vi "Configure Device.vi"(8 "error in":errorcluster, 11 "Alicat Device In":refnum<class "Alicat Device.lvclass">) -> (0 "error out":errorcluster, 3 "Alicat Device Out":refnum<class "Alicat Device.lvclass">, 4 "SP":dbl, 5 "Settable?":bool)   [LabVIEW 2014, in "Alicat Lib.lvlib" / "Alicat Device.lvclass"]
doc: "Configure the serial port for communication with the Alicat devices. We will create new Alicat objects based upon an input array of addresses. If an address is no good, then we will delete the session reference and move onto the next address. We determine if the session is good by sending a request for data to the device until the device \"wakes up\" and responds properly. If the device does not repsond properly, then set the boolean property <b>Active</b> to alert potential callers that this instantiation is non-communicative.\n\nAlthough the caller can configure the port with the desired serial and message settings, the default settings should be sufficient for most applications."
uses:
  Alicat Device.lvclass
  reusable/Session APIs/Serial/Serial Session.lvclass
  Data/Alicat Data.lvclass
  Configurable Device/Configurable Device.lvclass/Configurable Device.ctl
  reusable/Data/Data.lvclass/Data.ctl
  Data/Alicat Data.lvclass/Alicat Data.ctl
  Alicat Device.lvclass/Alicat Device.ctl
  reusable/Session APIs/File Access/Config Data/Config Data.lvclass/Config Data.ctl
  Configurable Device/Accessors/Write label.vi
  Accessors/Read Session Handle.vi
  Configurable Device/Read controller_.vi
  Accessors/Write Session Handle.vi
  Configurable Device/Accessors/Write type.vi
  reusable/Data/Write Data ID.vi
  Data/Accessors/Write ID.vi
  Configurable Device/Read Handle.vi
  Configurable Device/Read Log Session.vi
  <vilib>/Utility/config.llb/Read Key (String).vi
  <vilib>/Utility/config.llb/Read Key (Double).vi
  Configurable Device/Configurable Device.lvclass
  reusable/Session APIs/File Access/Config Data/Config Data.lvclass
  <userlib>/_Session Fwk/Session - Root.lvclass
  <vilib>/ErrorRing/Error Ring.xnode
  <vilib>/Utility/config.llb/NI_LVConfig.lvlib
  reusable/Session APIs/Session Log/System Log.lvclass
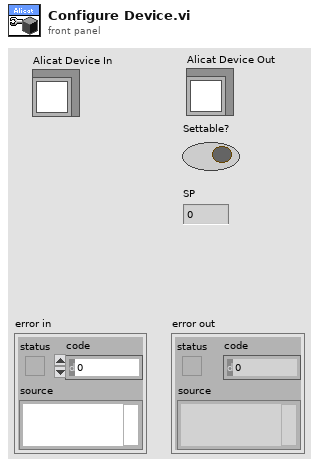
[diagram p1: front panel]
types:
  T1 = typedef "Serial Session.lvclass/Session Handle.ctl" = refnum<data-value>
  T2 = typedef "Config Data.lvclass/Config Session.ctl" = refnum<data-value>
  T3 = typedef "Session - Root.lvclass/Session Handle.ctl" = refnum<data-value>
  T4 = typedef "NI_LVConfig.lvlib/Config Data RefNum.ctl" = refnum<k1>
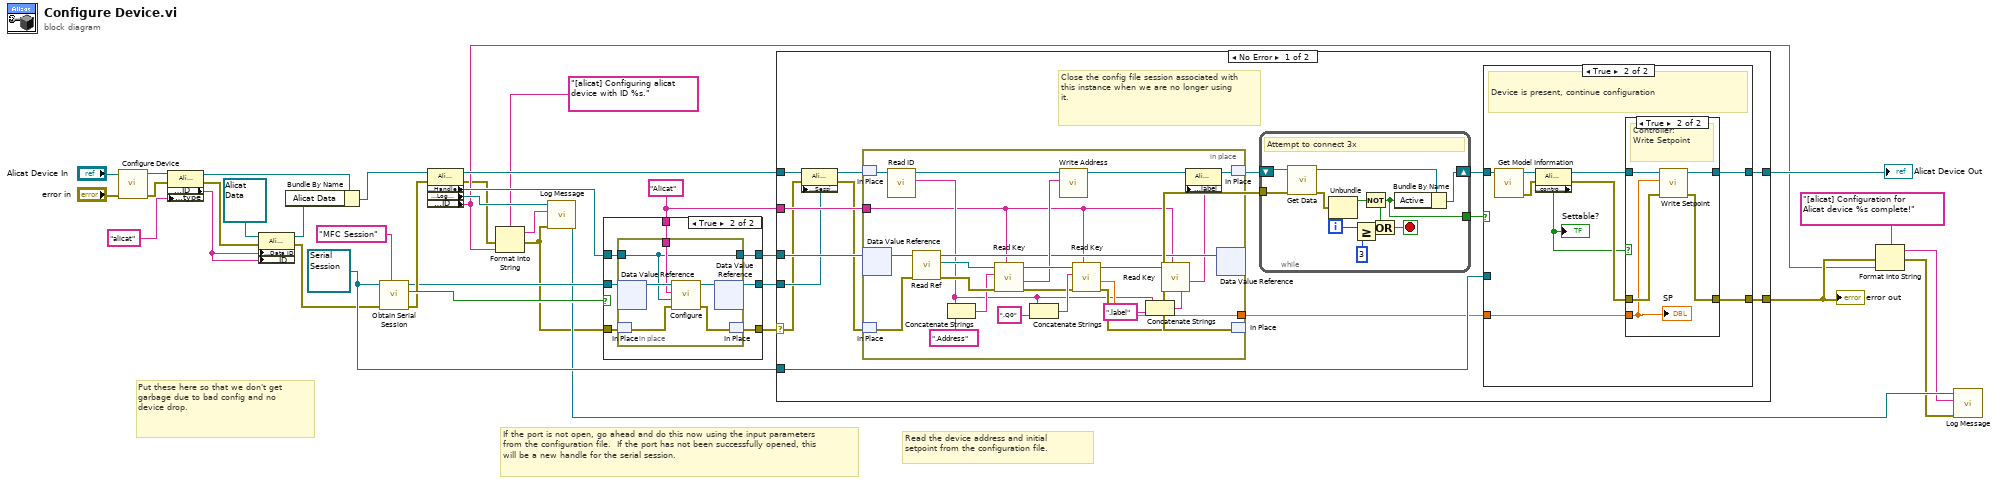
[diagram p0: block diagram]
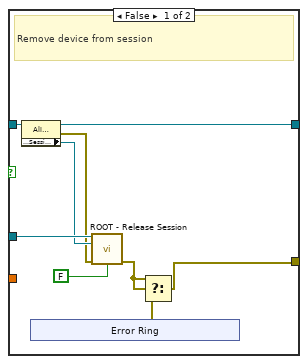
[diagram p2: hidden frame]
diagram:
  w28 = refnum<class "Serial Session.lvclass"> refnum ("Serial Session in")
  w30 = "Alicat" ("section")
  # "Put these here so that we don't get garbage due to bad config and no device drop."
  # "If the port is not open, go ahead and do this now using the input parameters from the configuration file.  If the port has not been successfully opened, this will be a new handle for the serial session."
  # "Read the device address and initial setpoint from the configuration file."
  n1 = call-parent "Configure Device.vi"("error in"="error in", "Device in"="Alicat Device In") -> ("error out"=w2:errorcluster, "Device out"=w3:refnum<class "Alicat Device.lvclass">)  [unwired: 6 in, 2 out]
  n2 = property class="Alicat Device"(reference=w3, error in=w2, "Accessors:type"="alicat" ("type")) -> (reference out=w12:refnum<class "Alicat Device.lvclass">, error out=w9:errorcluster, "Accessors:ID"=w13:string)
  n3 = property class="Alicat Data"(reference=refnum<class "Alicat Data.lvclass"> refnum ("Alicat Lib.lvlib:Alicat Data"), error in=w9, "Accessors:Data ID"=w13, "Accessors:ID"=w13) -> (reference out=w10:refnum<class "Alicat Data.lvclass">, error out=w8:errorcluster)
  n4 = Bundle By Name(cluster=w12, "Alicat Data"=w10) -> (w11:refnum<class "Alicat Device.lvclass">)
  n5 = call "Obtain Serial Session.vi"("Session Name ()"="MFC Session", "error in"=w8, "Serial Session in"=w28) -> ("error out"=w32:errorcluster, "created new?"=w35:bool, "hSerial"=w29:T1)  [unwired: 6 in]
  n6 = property class="Alicat Device"(reference=w11, error in=w32) -> (reference out=w27:refnum<class "Alicat Device.lvclass">, error out=w7:errorcluster, "Accessors:Handle"=w33:T2, "Accessors:Log Session"=w23:T3, "Accessors:ID"=w15:string)
  n7 = Format Into String(format string="[alicat] Configuring alicat device with ID %s.", error in=w7, w15) -> (resulting string=w21:string, error out=w6:errorcluster)  [unwired: 1 in]
  n8 = call "Log Message.vi"("error in"=w6, "MSG In"=w21, "session in"=w23) -> ("session out"=w20:T3)  [unwired: 7 in, 1 out]
  n9 = case shown="True" w35 {
    tunnel: w29 -> [w38 w45]
    tunnel: w6 -> [w37 w41]
    tunnel: [w38 w44] -> w26
    tunnel: [w37 w43] -> w25
    tunnel: w33 -> [w36 w42]
    tunnel: [w36 w40] -> w31
    tunnel: w30 -> [_ w39]
    frame False {
    }
    frame True {
      n10 = in-place {
        in-place-border: w42 -> [w46]
        in-place-border: w39 -> [w47]
        in-place-border: [w46] -> w40
        n11 = in-place-dvr #1(w45) -> (w51:refnum<class "Serial Session.lvclass">)  [unwired: 1 out]
        n12 = in-place-match #2(w41) -> (w50:errorcluster)
        n13 = call "Configure.vi"("error in"=w50, "Config Handle"=w46, "section"=w47, "Serial Session in"=w51) -> ("error out"=w49:errorcluster, "Serial Session out"=w48:refnum<class "Serial Session.lvclass">)  [unwired: 6 in]
        n14 = in-place-dvr #1(w48) -> (w44:T1)  [unwired: 1 out]
        n15 = in-place-match #2(w49) -> (w43:errorcluster)
      }
    }
  }
  n16 = case shown="No Error" w25 {
    selector: w25 -> [w54 w128]
    tunnel: w31 -> [w66 _]
    tunnel: w30 -> [w65 _]
    tunnel: w28 -> [w64 _]
    tunnel: [w62 w128] -> w16
    tunnel: [w59 w129] -> w24
    tunnel: w27 -> [w58 w129]
    tunnel: w26 -> [w56 _]
    frame No Error {
      # "Close the config file session associated with this instance when we are no longer using it."
      n17 = property class="Alicat Device"(reference=w58, error in=w54, "Accessors:Session Handle"=w56) -> (reference out=w57:refnum<class "Alicat Device.lvclass">, error out=w55:errorcluster)
      n18 = in-place {
        in-place-border: w65 -> [w104]
        in-place-border: [w116] -> w60
        n19 = in-place-match #3(w57) -> (w114:refnum<class "Alicat Device.lvclass">)
        n20 = in-place-dvr #4(w66) -> (w127:refnum<class "Config Data.lvclass">)  [unwired: 1 out]
        n21 = in-place-match #5(w55) -> (w126:errorcluster)
        n22 = call "Read ID.vi"("Configurable Device in"=w114) -> ("ID"=w107:string, "Configurable Device out"=w113:refnum<class "Alicat Device.lvclass">)  [unwired: 8 in, 1 out]
        n23 = call "Read Ref.vi"("error in"=w126, "Config Data in"=w127) -> ("error out"=w124:errorcluster, "config data"=w125:T4, "Config Data out"=w115:refnum<class "Config Data.lvclass">)  [unwired: 7 in]
        n24 = Concatenate Strings(w107, ".Address" ("string")) -> (w122:string)
        n25 = call-poly <vilib>:"Read Key.vi"("section"=w104, "error in (no error)"=w124, "key"=w122, "refnum"=w125) -> ("error out"=w118:errorcluster, "value"=w117:string, "refnum out"=w121:T4)  [unwired: 4 in, 1 out]
        n26 = Concatenate Strings(w107, ".Q0" ("string")) -> (w119:string)
        n27 = call "Write Address.vi"("Address"=w117, "Alicat Device in"=w113) -> ("Alicat Device out"=w111:refnum<class "Alicat Device.lvclass">)  [unwired: 8 in, 1 out]
        n28 = call-poly <vilib>:"Read Key.vi"("section"=w104, "error in (no error)"=w118, "key"=w119, "refnum"=w121) -> ("error out"=w112:errorcluster, "value"=w116:dbl, "refnum out"=w106:T4)  [unwired: 4 in, 1 out]
        n29 = Concatenate Strings(w107, ".label" ("string")) -> (w108:string)
        n30 = call-poly <vilib>:"Read Key.vi"("section"=w104, "key"=w108, "refnum"=w106) -> ("value"=w105:string)  [unwired: 5 in, 3 out]
        n31 = property class="Alicat Device"(reference=w111, "Accessors:label"=w105) -> (reference out=w110:refnum<class "Alicat Device.lvclass">)  [unwired: 1 in, 1 out]
        n32 = in-place-dvr #4(w115) -> ()  [unwired: 2 out]
        n33 = in-place-match #3(w110) -> (w63:refnum<class "Alicat Device.lvclass">)
        n34 = in-place-match #5(w112) -> (w52:errorcluster)
      }
      n35 = while {
        tunnel: w52 -> [w98]
        shift-right: [w96] -> w61
        shift-left: w63 -> [w99]
        tunnel: [w95] -> w53
        i -> [w93]
        stop <- w100 stop-if-true
        # "Attempt to connect 3x"
        n36 = call-dynamic "Get Data.vi"("error in"=w98, "Alicat Device in"=w99) -> ("error out"=w94:errorcluster, "Alicat Device out"=w97:refnum<class "Alicat Device.lvclass">)  [unwired: 7 in, 1 out]
        n37 = Unbundle(w94) -> ("status"=w101:bool)  [unwired: 2 out]
        n38 = Greater Or Equal?(x=w93, y=3) -> (x >= y?=w102:bool)
        n39 = Not(x=w101) -> (.not. x?=w95:bool)
        n40 = Or(x=w95, y=w102) -> (x .or. y?=w100:bool)
        n41 = Bundle By Name(cluster=w97, "Active"=w95) -> (w96:refnum<class "Alicat Device.lvclass">)
      }
      n42 = case shown="True" w53 {
        tunnel: [w67 w83] -> w62
        tunnel: w64 -> [w75 _]
        tunnel: w61 -> [w73 w85]
        tunnel: w60 -> [_ w84]
        tunnel: [w72 w82] -> w59
        frame False {
          # "Remove device from session"
          n43 = property class="Alicat Device"(reference=w73) -> (reference out=w72:refnum<class "Alicat Device.lvclass">, error out=w70:errorcluster, "Accessors:Session Handle"=w71:T1)  [unwired: 1 in]
          n44 = xnode "Error Ring"() -> ("error out"=w68:errorcluster)
          n45 = call <userlib>:"ROOT - Release Session.vi"("OBJ - Session in"=w75, "Session Handle in"=w71, "error in (no error)"=w70, "force destroy? (F)"=FALSE) -> ("error out"=w69:errorcluster)  [unwired: 10 in, 1 out]
          n46 = Select(t=w69, s=w69, f=w68) -> (s? t:f=w67:errorcluster)
        }
        frame True {
          # "Device is present, continue configuration"
          n47 = call "Get Model Information.vi"("Alicat Device in"=w85) -> ("error out"=w77:errorcluster, "Alicat Device out"=w81:refnum<class "Alicat Device.lvclass">)  [unwired: 7 in, 2 out]
          n48 = property class="Alicat Device"(reference=w81, error in=w77) -> (reference out=w80:refnum<class "Alicat Device.lvclass">, error out=w79:errorcluster, "Accessors:controller_"=w78:bool)
          "Settable?" <- w78
          n49 = case shown="True" w78 {
            tunnel: w79 -> [w86 w91]
            tunnel: w80 -> [w87 w92]
            tunnel: w84 -> [_ w88]
            tunnel: [w86 w90] -> w83
            tunnel: [w87 w89] -> w82
            frame False {
            }
            frame True {
              # "Controller:\nWrite Setpoint"
              n50 = call "Write Setpoint.vi"("error in"=w91, "Setpoint"=w88, "Alicat Device in"=w92) -> ("error out"=w90:errorcluster, "Alicat Device out"=w89:refnum<class "Alicat Device.lvclass">)  [unwired: 6 in, 1 out]
              "SP" <- w88
            }
          }
        }
      }
    }
    frame Error {
    }
  }
  "error out" <- w16
  "Alicat Device Out" <- w24
  n51 = Format Into String(format string="[alicat] Configuration for Alicat device %s complete!", error in=w16, w15) -> (resulting string=w18:string, error out=w17:errorcluster)  [unwired: 1 in]
  n52 = call "Log Message.vi"("error in"=w17, "MSG In"=w18, "session in"=w20) -> ()  [unwired: 7 in, 2 out]
